vi "Q-3.vi"(0 "Application_Directory":path, 11 "Error_In":errorcluster) -> (15 "Error_Out":errorcluster)   [LabVIEW 2021]
doc: "This is a VI works as one of the front panel of the Game asking the user the third question."
uses:
  Controls/State.ctl
  Controls/Bool_Button.ctl
panel:
  in  "Home":T1=TRUE
  in  "Back?":T1=TRUE
  in  "Place_Option":T2(ring) caption="Select the Place"
  # "Do you like \n‘sea’, ‘ocean’, ‘mountains"
  # "Excellent choice! Now, to further refine the magic that will reveal your destiny, I must ask you one more question"
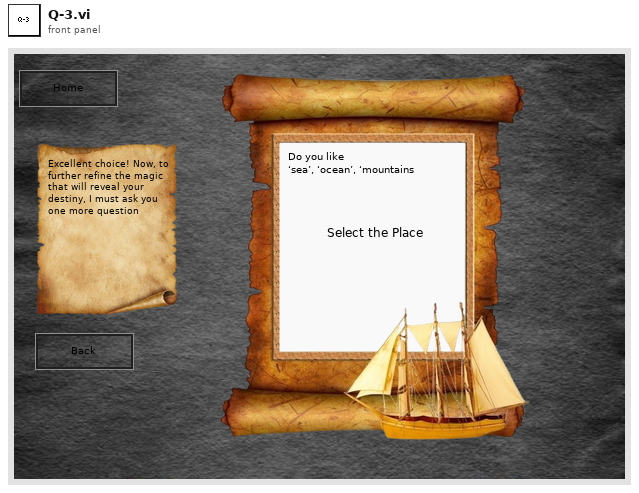
[diagram p1: front panel]
types:
  T1 = typedef "Bool_Button.ctl" = bool
  T2 = enum16{"Select the Place", "Sea", "Ocean", "Mountains"}
  T3 = enum32{"Invalid", "Standard", "Closed", "Hidden", "Minimized", "Maximized"}
  T4 = typedef "State.ctl" = enum16{"Close", "Password_Popup", "Start_Popup", "Wizard_Msg", "Get_Name_DoB", "Lucky_Number", "Q-1", "Q-2", "Q-3", "Nature_of_the_Person"}
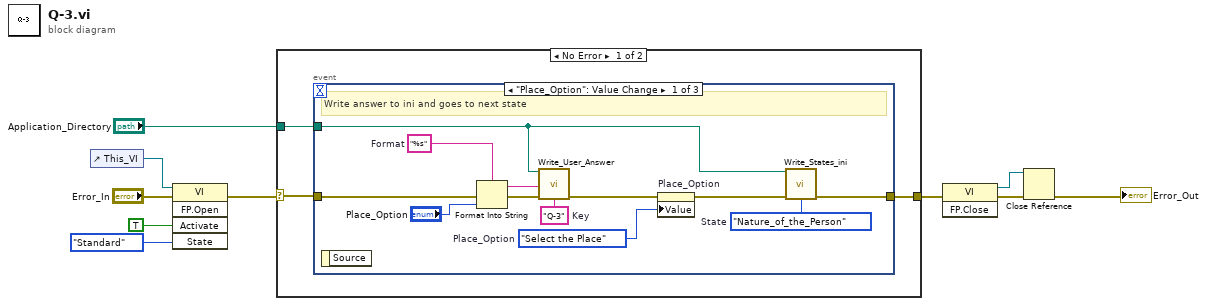
[diagram p0: block diagram]
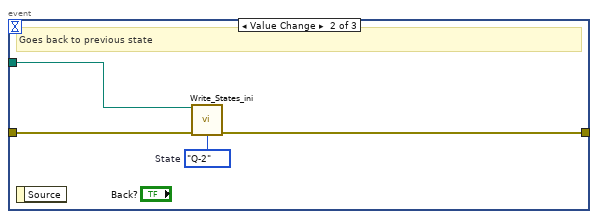
[diagram p2: hidden frame]
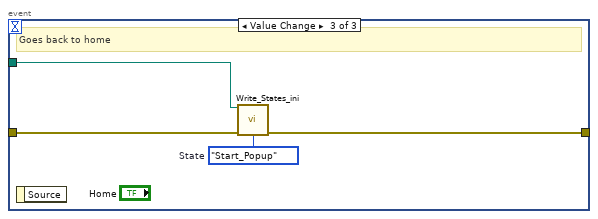
[diagram p3: hidden frame]
diagram:
  n1 = control-ref of="This_VI"() -> (w8:refnum<vi>)
  n2 = invoke class="VI" method="FP.Open"(reference=w8, error in="Error_In", "Activate"=TRUE ("Activate?"), "State"=T3."Standard") -> (error out=w9:errorcluster)  [unwired: 1 in, 4 out]
  n3 = case shown="No Error" w9 {
    selector: w9 -> [w13 w34]
    tunnel: [w12 w34] -> w4
    tunnel: "Application_Directory" -> [w11 _]
    frame No Error {
      n4 = event shown="[0] \"Place_Option\": Value Change" {
        selector: _ -> [_ _ _]
        dyn-events: _ -> [_ _ _]
        timeout: _ -> [_ _ _]
        tunnel: w13 -> [w24 w29 w33]
        tunnel: [w21 w28 w32] -> w12
        tunnel: w11 -> [w19 w27 w30]
        event "Place_Option": Value Change {
          w14 = "Q-3"  # Key
          w20 = State."Nature_of_the_Person"  # State
          w22 = T2."Select the Place"  # Place_Option
          w23 = "%s"  # Format
          # "Write answer to ini and goes to next state"
          n5 = event-data() -> ()  [unwired: 1 in, 1 out]
          n6 = Format Into String(format string=w23, error in=w24, "Place_Option") -> (resulting string=w16:string, error out=w17:errorcluster)  [unwired: 1 in]
          n7 = call "Write_User_Answer.vi"("Application_Directory"=w19, "Data"=w16, "Error_In"=w17, "Key"=w14) -> ("Error_Out"=w18:errorcluster)  [unwired: 11 in]
          n8 = property on="Place_Option" class="Enum (strict)"(error in=w18, "Value"=w22) -> (error out=w15:errorcluster)  [unwired: 1 in, 1 out]
          n9 = call "Write_States_ini.vi"("Application_Directory"=w19, "Error_In"=w15, "State"=w20) -> ("Error_Out"=w21:errorcluster)  [unwired: 12 in]
        }
        event Value Change {
          w26 = State."Q-2"  # State
          # "Goes back to previous state"
          n10 = event-data() -> ()  [unwired: 1 in, 1 out]
          n11 = call "Write_States_ini.vi"("Application_Directory"=w27, "Error_In"=w29, "State"=w26) -> ("Error_Out"=w28:errorcluster)  [unwired: 12 in]
        }
        event Value Change {
          w31 = State."Start_Popup"  # State
          # "Goes back to home"
          n12 = event-data() -> ()  [unwired: 1 in, 1 out]
          n13 = call "Write_States_ini.vi"("Application_Directory"=w30, "Error_In"=w33, "State"=w31) -> ("Error_Out"=w32:errorcluster)  [unwired: 12 in]
        }
      }
    }
    frame Error {
    }
  }
  n14 = invoke class="VI" method="FP.Close"(error in=w4) -> (reference out=w5:refnum<vi>, error out=w6:errorcluster)  [unwired: 2 in, 1 out]
  n15 = Close Reference(reference=w5, error in (no error)=w6) -> (error out=→"Error_Out":errorcluster)
